vi "test-PID-test-03-OnTargetNoToleranceSet.vi"() -> (3 "All Passed":bool)   [LabVIEW 2019]
uses:
  <vilib>/Rock Robotics/WPI/ThirdParty/JAS_Junk/TrajLib/ControllerUtil_GetModulusError.vi
  <vilib>/Rock Robotics/WPI/ThirdParty/JAS_Junk/TrajLib/Trajectory_Library.lvlib
panel:
  out "AtSetpoint":bool
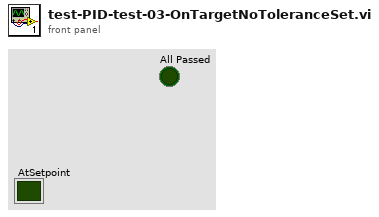
[diagram p1: front panel]
types:
  T1 = typedef "Trajectory_Library.lvlib/PID_CONTROLLER.ctl" = cluster{"Kp":dbl, "Ki":dbl, "Kd":dbl, "Period":dbl, "Max_Integral":dbl, "Min_Integral":dbl, "Max_Input":dbl, "Min_Input":dbl, "Continuous":bool, "PositionError":dbl, "VelocityError":dbl, "PrevError":dbl, "TotalError":dbl, "PositionTolerance":dbl, "VelocityTolerance":dbl, "SetPoint":dbl, "Kf":dbl, "Prev_Deriv":dbl, "Prev_Deriv 2":dbl, "DerivativeFilter":bool, "Min_Output":dbl, "Max_Output":dbl, "Prev_F_P":dbl, "Prev_F_P_2":dbl, "AntiWindupActive":bool, "Measurement":dbl}
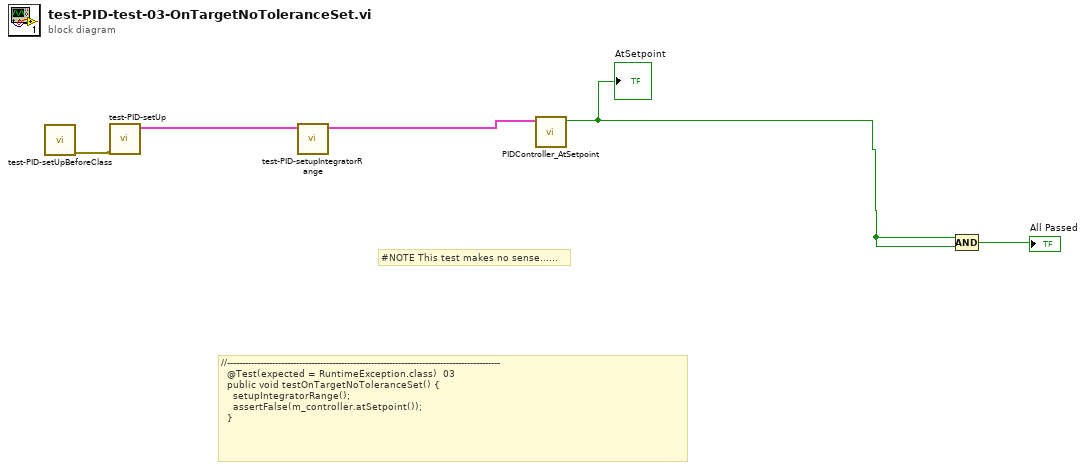
[diagram p0: block diagram]
diagram:
  # "#NOTE This test makes no sense......"
  # "//-------------------------------------------------------------------------------------------\n  @Test(expected = RuntimeException.class)  03\n  public void testOnTargetNoToleranceSet() {\n    setupIntegratorRange();\n    assertFalse(m_controller.atSetpoint());\n  }"
  n1 = call "test-PID-setUpBeforeClass.vi"() -> ("error out"=w5:errorcluster)  [unwired: 11 in]
  n2 = call "test-PID-setUp.vi"("error in (no error)"=w5) -> ("PID_CONTROLLER"=w3:T1)  [unwired: 9 in, 1 out]
  n3 = call "test-PID-setupIntegratorRange.vi"("in PID_CONTROLLER"=w3) -> ("out PID_CONTROLLER"=w2:T1)  [unwired: 10 in]
  n4 = call <vilib>:"PIDController_AtSetpoint.vi"("in PID_CONTROLLER"=w2) -> ("AtSetpoint"=w1:bool)  [unwired: 10 in]
  "AtSetpoint" <- w1
  n5 = Compound Arithmetic op=AND(w1, w1) -> (→"All Passed":bool)
